vi "Get divisors-test harness.vi"(8 "error in (no error)":errorcluster) -> (0 "error out":errorcluster)   [LabVIEW 2021, in "Numeric Utilities.lvlib"]
uses:
  Numeric Utilities.lvlib
panel:
  out "Loop 2":i32
  out "Loop 1":i32
  in  "Dev: Stop early":bool
  out "power set (seconds)":dbl
  out "exhaustive enumeration (seconds)":dbl
  out "Test vector":i32[](array[numeric])
  in  "Offset":i32=1
  in  "Number of integers to test with":i32=1000000
  # "Development\ncontrols/indicators useful for development and testing, but which are not outputs of the VI"
  # "Input\nInputs to the VI"
  # "Output\nOutputs of the VI"
  # "Description\n\nBlank VI with error handling case. \n\nSummarize the use of this VI in this space."
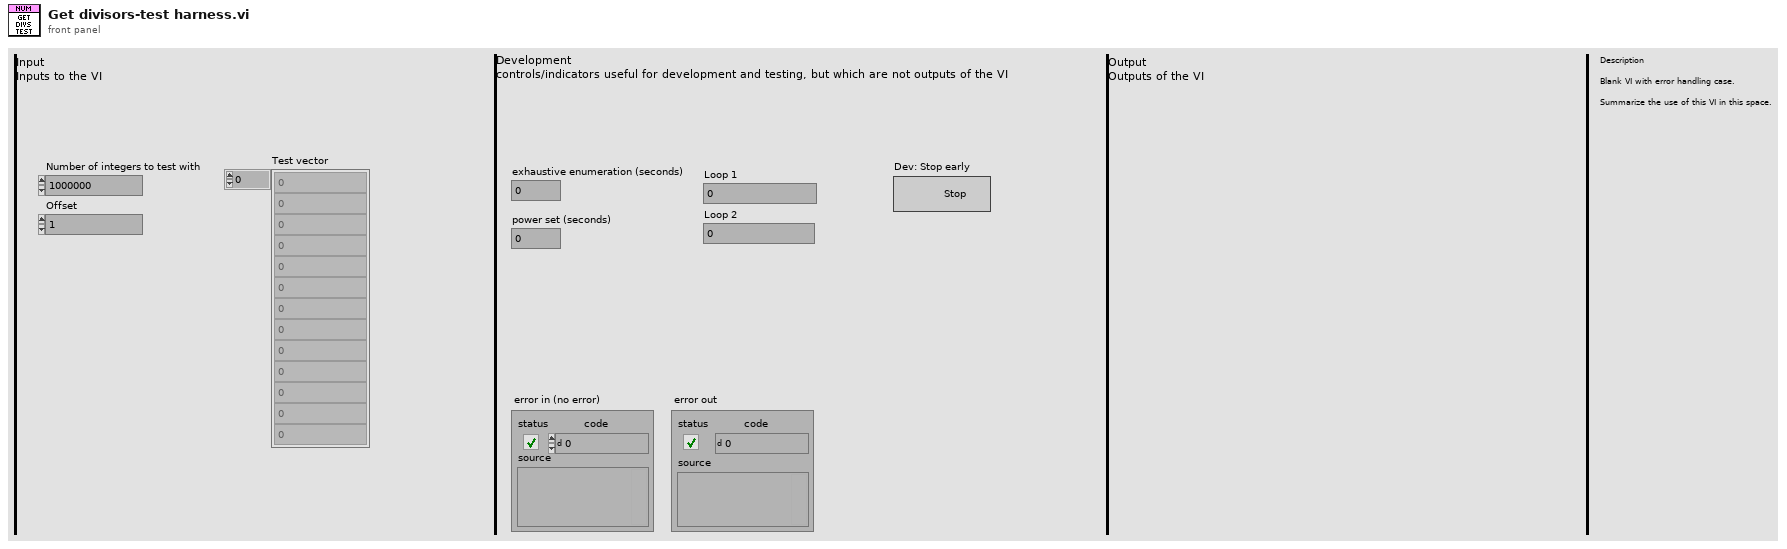
[diagram p1: front panel]
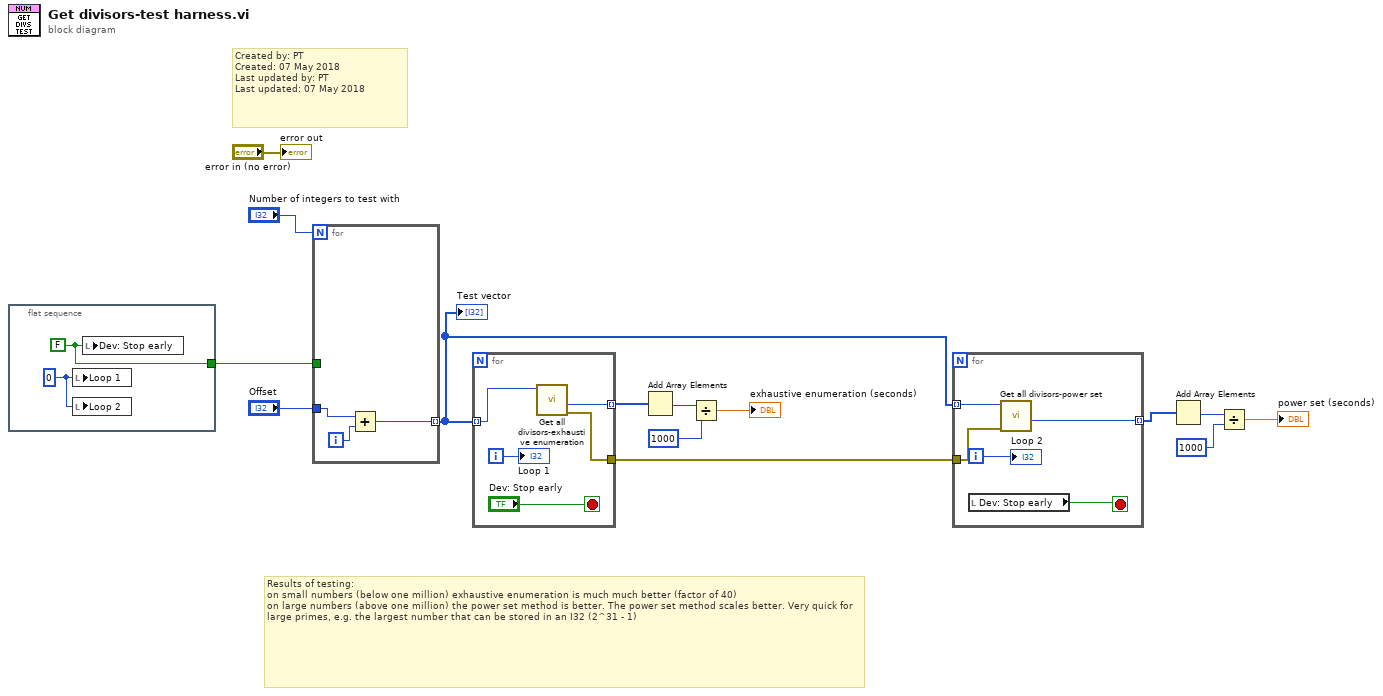
[diagram p0: block diagram]
diagram:
  # "Results of testing:\non small numbers (below one million) exhaustive enumeration is much much better (factor of 40)\non large numbers (above one million) the power set method is better. The power set method scales better. Very quick for large primes, e.g. the largest number that can be stored in an I32 (2^31 - 1)"
  # "Created by: PT\nCreated: 07 May 2018\nLast updated by: PT\nLast updated: 07 May 2018"
  n1 = flat-sequence {
    tunnel: [w16] -> w1
    frame #0 {
      w15 = 0 ("Loop 1")
      w16 = FALSE ("Dev: Stop early")
      n2 = local write "Loop 1"(w15) -> ()
      n3 = local write "Loop 2"(w15) -> ()
      n4 = local write "Dev: Stop early"(w16) -> ()
    }
  }
  n5 = for {
    N: "Number of integers to test with" -> [_]
    tunnel: "Offset" -> [w19]
    tunnel: [w17] -> w7 mode=indexing
    tunnel: w1 -> [_]
    i -> [w18]
    n6 = Add(x=w19, y=w18) -> (x+y=w17:i32)
  }
  "Test vector" <- w7
  n7 = for {
    tunnel: w7 -> [w24] mode=indexing
    tunnel: [w23] -> w11 mode=indexing
    tunnel: [w22] -> w6
    i -> [w21]
    stop <- "Dev: Stop early" stop-if-true
    n8 = call "Get all divisors-exhaustive enumeration.vi"("x"=w24) -> ("error out"=w22:errorcluster, "Execution time (ms)-Total"=w23:u32)  [unwired: 7 in, 2 out]
    "Loop 1" <- w21
  }
  n9 = Add Array Elements(numeric array=w11) -> (sum=w10:u32)
  n10 = Divide(x=w10, y=u32 1000) -> (x/y=→"exhaustive enumeration (seconds)":dbl)
  n11 = for {
    tunnel: w7 -> [w29] mode=indexing
    tunnel: w6 -> [w28]
    tunnel: [w27] -> w3 mode=indexing
    i -> [w26]
    stop <- w25 stop-if-true
    n12 = local read "Dev: Stop early"() -> (w25:bool)
    n13 = call "Get all divisors-power set.vi"("error in (no error)"=w28, "x"=w29) -> ("Execution time (ms)-Total"=w27:u32)  [unwired: 6 in, 3 out]
    "Loop 2" <- w26
  }
  n14 = Add Array Elements(numeric array=w3) -> (sum=w4:u32)
  n15 = Divide(x=w4, y=u32 1000) -> (x/y=→"power set (seconds)":dbl)
  "error out" <- "error in (no error)"
